vi "BMP to 2D Array.vi"(4 "BMP image data":T1) -> (1 "2D pixel array":u32[][](array[numeric]))   [LabVIEW 2013]
uses:
  <vilib>/picture/picture.llb/imagedata.ctl
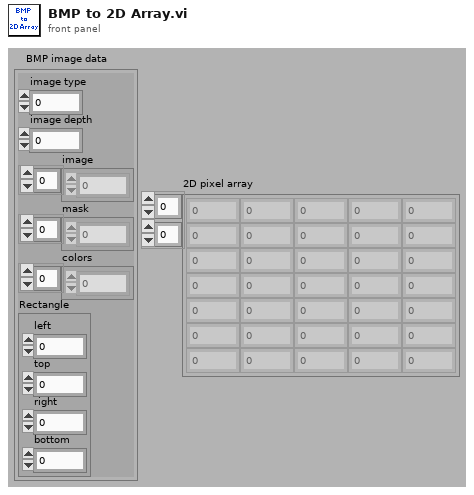
[diagram p1: front panel]
types:
  T1 = typedef "imagedata.ctl" = cluster{"image type":i32, "image depth":i32, "image":u8[], "mask":u8[], "colors":u32[], "Rectangle":cluster{"left":i16, "top":i16, "right":i16, "bottom":i16}}
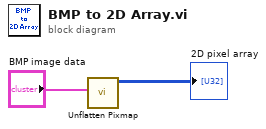
[diagram p0: block diagram]
diagram:
  n1 = call <vilib>:"Unflatten Pixmap.vi"("image data"="BMP image data") -> ("24-bit pixmap"=→"2D pixel array":u32[][])  [unwired: 4 in, 6 out]
